vi "Save for 2020.vi"   [LabVIEW 2023]
panel:
  # "Run me to populate the folder"
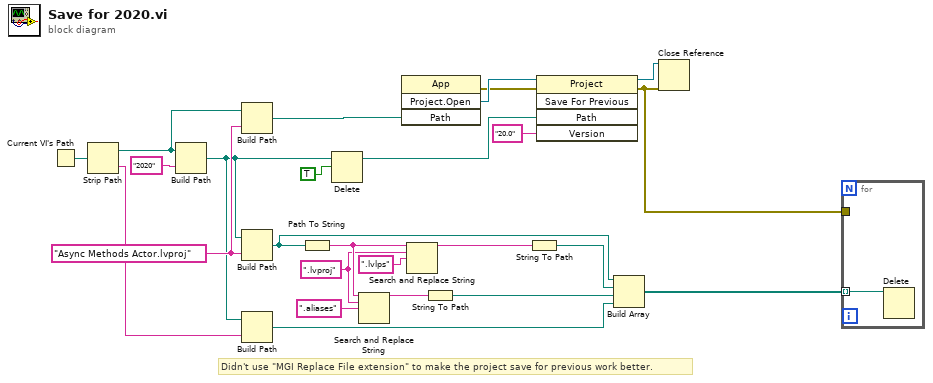
[diagram p0: block diagram]
diagram:
  w4 = ".lvproj" ("search string")
  w16 = "Async Methods Actor.lvproj" ("name or relative path")
  # "Didn't use \"MGI Replace File extension\" to make the project save for previous work better."
  n1 = Current VI's Path() -> (path=w25:path)
  n2 = Strip Path(path=w25) -> (stripped path=w2:path, name=w15:string)
  n3 = Build Path(base path=w2, name or relative path="2020") -> (appended path=w1:path)
  n4 = Build Path(base path=w2, name or relative path=w16) -> (appended path=w19:path)
  n5 = Build Path(base path=w1, name or relative path=w16) -> (appended path=w10:path)
  n6 = Build Path(base path=w1, name or relative path=w15) -> (appended path=w14:path)
  n7 = Path To String(path=w10) -> (string=w7:string)
  n8 = Delete(path (use dialog)=w1, entire hierarchy (F)=TRUE) -> (deleted path=w23:path)  [unwired: 3 in, 2 out]
  n9 = Search and Replace String(input string=w7, search string=w4, replace string=".aliases" ("replace string (\"\")")) -> (result string=w6:string)  [unwired: 5 in, 3 out]
  n10 = invoke class="App" method="Project.Open"("Path"=w19) -> (error out=w17:errorcluster, "Project:Open"=w20:refnum<vi>)  [unwired: 3 in, 2 out]
  n11 = Search and Replace String(input string=w7, search string=w4, replace string=".lvlps" ("replace string (\"\")")) -> (result string=w9:string)  [unwired: 5 in, 3 out]
  n12 = String To Path(string=w6) -> (path=w5:path)
  n13 = String To Path(string=w9) -> (path=w8:path)
  n14 = invoke class="Project" method="Save For Previous"(reference=w20, error in=w17, "Path"=w23, "Version"="20.0") -> (reference out=w18:refnum<vi>, error out=w12:errorcluster)  [unwired: 1 in, 3 out]
  n15 = Build Array(w10, w8, w5, w14) -> (w13:path[])
  n16 = Close Reference(reference=w18, error in (no error)=w12) -> ()  [unwired: 1 out]
  n17 = for {
    tunnel: w13 -> [w26] mode=indexing
    tunnel: w12 -> [_]
    n18 = Delete(path (use dialog)=w26) -> ()  [unwired: 4 in, 3 out]
  }
